vi "Remove Node RecursiveChild.vi"(10 "New Node Path (parent, child)":string[](array[string]), 11 "Tree Map In":T1) -> (0 "error out":errorcluster, 2 "Node removed?":bool, 3 "Tree Map Out":T1)   [LabVIEW 2020, in "Blue Tree Map OpenSource.lvlib"]
uses:
  Blue Tree Map OpenSource.lvlib
  Typedefs/Tree Map.ctl
  Typedefs/Tree Map Data.ctl
  Typedefs/Tree Node Data.ctl
  Typedefs/Attribute Map.ctl
  <vilib>/Utility/miscctls.llb/LVMapReplaceAction.ctl
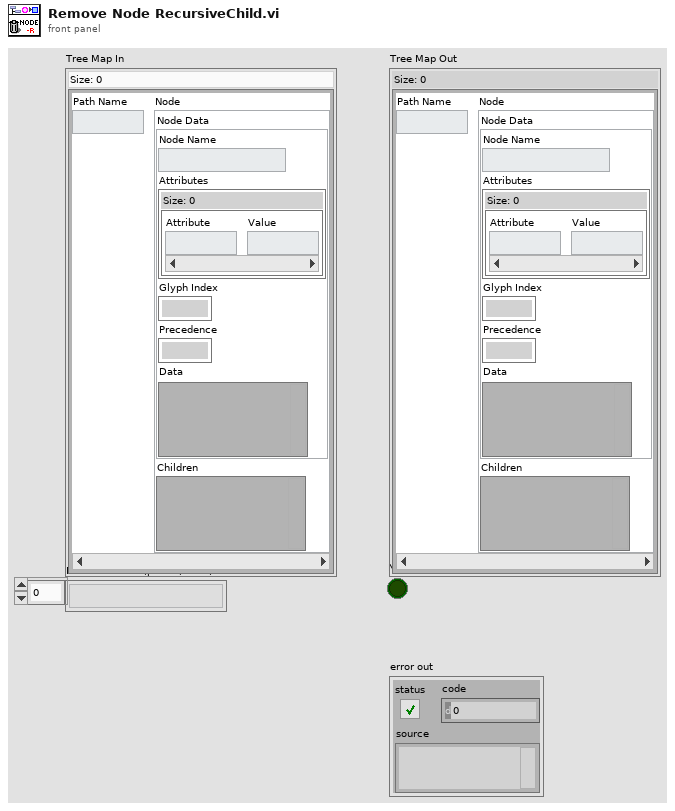
[diagram p1: front panel]
types:
  T1 = typedef "Blue Tree Map OpenSource.lvlib/Tree Map.ctl" = map{string, T2}
  T2 = typedef "Blue Tree Map OpenSource.lvlib/Tree Map Data.ctl" = cluster{"Node Data":T3, "Children":variant}
  T3 = typedef "Blue Tree Map OpenSource.lvlib/Tree Node Data.ctl" = cluster{"Node Name":string, "Attributes":T4, "Glyph Index":i32, "Precedence":i32, "Data":variant}
  T4 = typedef "Blue Tree Map OpenSource.lvlib/Attribute Map.ctl" = map{string, string}
  T5 = typedef "LVMapReplaceAction.ctl" = enum32{"Modify Entry only if found", "Add or Modify Entry", "Delete Entry"}
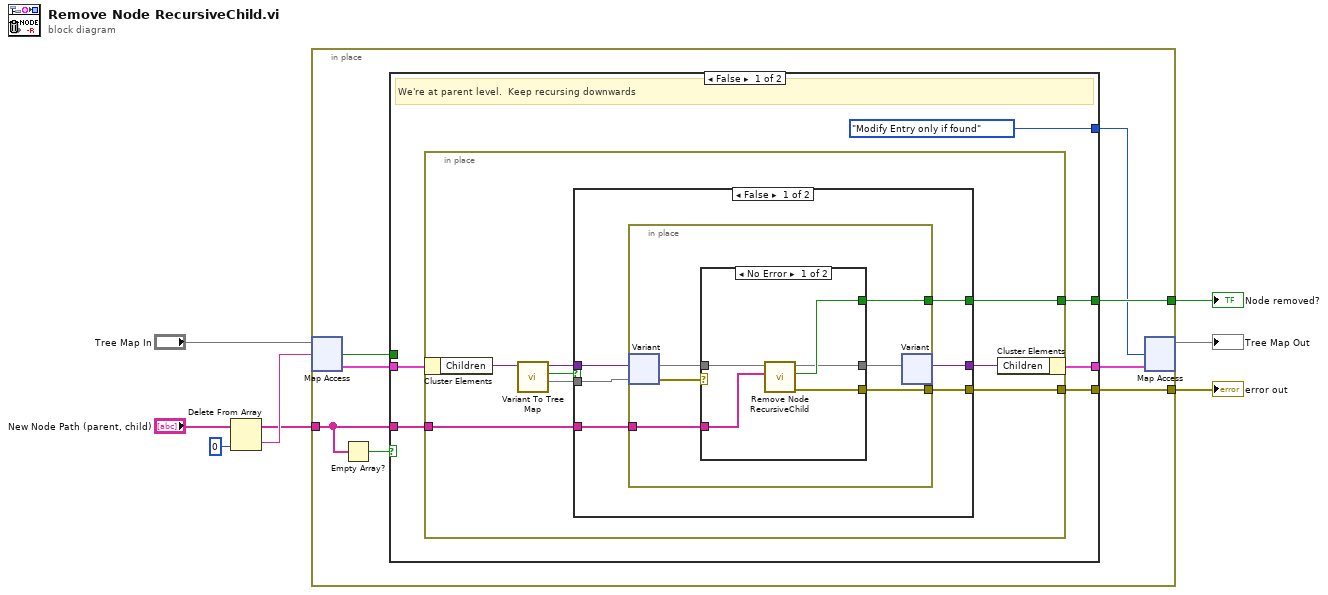
[diagram p0: block diagram]
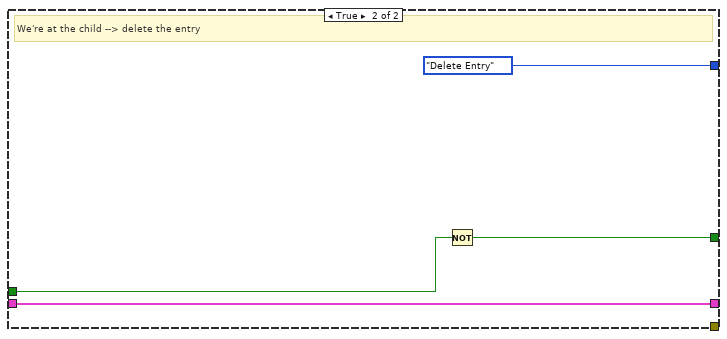
[diagram p4: hidden frame]
diagram:
  n1 = Delete From Array(array="New Node Path (parent, child)", index=0) -> (deleted portion=w2:string, array with subset deleted=w1:string[])  [unwired: 1 in]
  n2 = in-place {
    in-place-border: w1 -> [w9]
    in-place-border: [w15] -> w7
    in-place-border: [w13] -> w6
    n3 = in-place-map #1("Tree Map In", w2) -> (w16:T2, w11:bool)  [unwired: 1 in]
    n4 = Empty Array?(array=w9) -> (empty?=w10:bool)
    n5 = case shown="False" w10 {
      tunnel: w16 -> [w22 w51]
      tunnel: w9 -> [w21 _]
      tunnel: [w20 _] -> w15
      tunnel: [w19 w51] -> w14
      tunnel: [w18 w53] -> w13
      tunnel: [LVMapReplaceAction."Modify Entry only if found" ("action") LVMapReplaceAction."Delete Entry" ("action")] -> w12
      tunnel: w11 -> [_ w52]
      frame False {
        # "We're at parent level.  Keep recursing downwards"
        n6 = in-place {
          in-place-border: w21 -> [w29]
          in-place-border: [w28] -> w20
          in-place-border: [w27] -> w18
          n7 = in-place-cluster #2(w22) -> ("Children"=w30:variant)
          n8 = call "Variant To Tree Map.vi"("Children"=w30) -> ("Tree Map (Empty)"=w25:T1, "Empty?"=w24:bool, "Children"=w26:variant)  [unwired: 8 in]
          n9 = case shown="False" w24 {
            tunnel: w29 -> [w36 _]
            tunnel: [w35 _] -> w28
            tunnel: [w34 _] -> w27
            tunnel: w26 -> [w33 w50]
            tunnel: w25 -> [w32 _]
            tunnel: [w31 w50] -> w23
            frame False {
              n10 = in-place {
                in-place-border: w36 -> [w42]
                in-place-border: [w41] -> w35
                in-place-border: [w40] -> w34
                n11 = in-place-variant #3(w33, w32) -> (w39:T1, w37:errorcluster)
                n12 = case shown="No Error" w37 {
                  selector: w37 -> [_ w48]
                  tunnel: w42 -> [w47 _]
                  tunnel: [w46 w48] -> w41
                  tunnel: [w45 _] -> w40
                  tunnel: w39 -> [w44 w49]
                  tunnel: [w43 w49] -> w38
                  frame No Error {
                    n13 = call "Remove Node RecursiveChild.vi"("New Node Path (parent, child)"=w47, "Tree Map In"=w44) -> ("error out"=w46:errorcluster, "Node removed?"=w45:bool, "Tree Map Out"=w43:T1)  [unwired: 7 in]
                  }
                  frame Error {
                  }
                }
                n14 = in-place-variant #3(w38) -> (w31:variant)  [unwired: 1 out]
              }
            }
            frame True {
            }
          }
          n15 = in-place-cluster #2("Children"=w23) -> (w19:T2)
        }
      }
      frame True {
        # "We're at the child --> delete the entry"
        n16 = Not(x=w52) -> (.not. x?=w53:bool)
      }
    }
    n17 = in-place-map #1(w14, w12) -> (→"Tree Map Out":T1)  [unwired: 2 out]
  }
  "error out" <- w7
  "Node removed?" <- w6
